vi "CAN BL Set New Baud Rate.vi"(5 "TimeOut":u32, 6 "NewBaudRate":u32, 7 "pInitConfig":T1, 9 "NodeAddr":u16, 10 "CANIndex":i32, 11 "DevHandle":i32) -> (2 "function return":i32, 3 "pInitConfig out":T1)   [LabVIEW 2010, in "usb2can.lvlib"]
doc: "int WINAPI CAN_BL_SetNewBaudRate(int DevHandle,int CANIndex,unsigned short NodeAddr,CAN_INIT_CONFIG *pInitConfig,unsigned int NewBaudRate,unsigned int TimeOut);"
uses:
  usb2can.lvlib
  USB2XXX/trunk/USB2XXX/USB2XXX/vs2019/Release/USB2XXX.dll
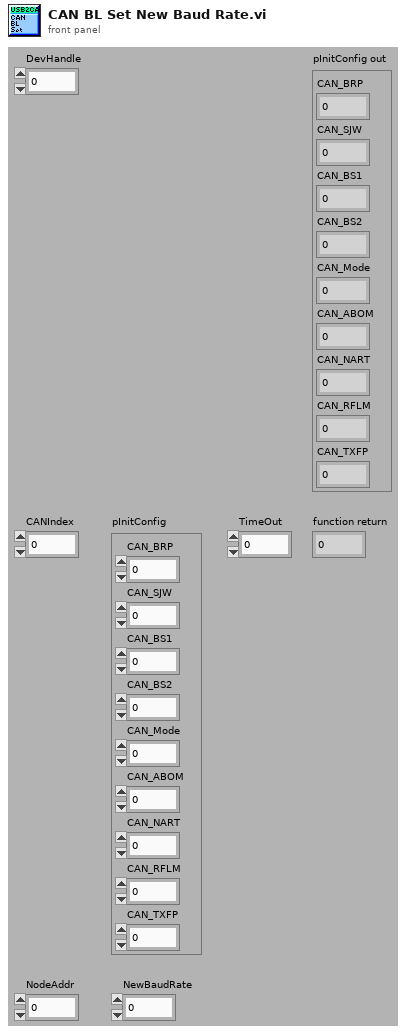
[diagram p1: front panel]
types:
  T1 = cluster{"CAN_BRP":u32, "CAN_SJW":u8, "CAN_BS1":u8, "CAN_BS2":u8, "CAN_Mode":u8, "CAN_ABOM":u8, "CAN_NART":u8, "CAN_RFLM":u8, "CAN_TXFP":u8}
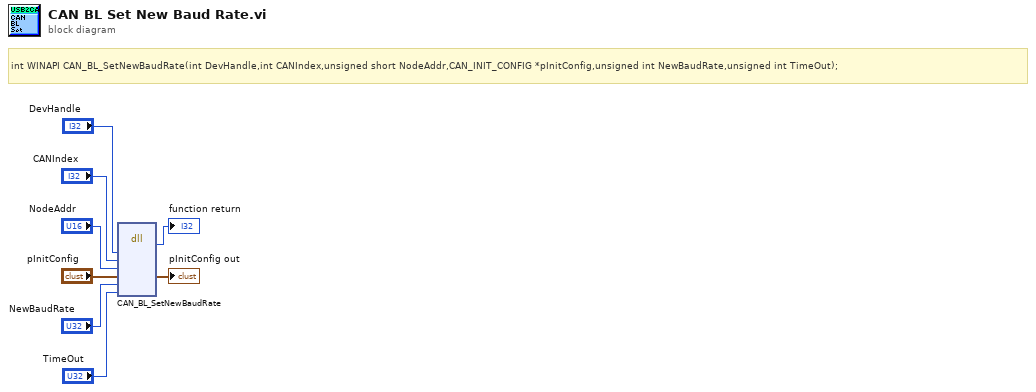
[diagram p0: block diagram]
diagram:
  # "int WINAPI CAN_BL_SetNewBaudRate(int DevHandle,int CANIndex,unsigned short NodeAddr,CAN_INIT_CONFIG *pInitConfig,unsigned int NewBaudRate,unsigned int TimeOut);"
  n1 = dll-call lib="E:/Projects/USB2XXX/trunk/USB2XXX/USB2XXX/vs2019/Release/USB2XXX.*" fn="CAN_BL_SetNewBaudRate"("DevHandle"="DevHandle", "CANIndex"="CANIndex", "NodeAddr"="NodeAddr", "pInitConfig"="pInitConfig", "NewBaudRate"="NewBaudRate", "TimeOut"="TimeOut") -> (→"function return":i32, "pInitConfig"=→"pInitConfig out":T1)  [unwired: 8 in, 2 out]
